vi "Get LabVIEW Install Paths.vi"(8 "Error In":errorcluster) -> (0 "Error Out":errorcluster, 2 "LV Directories":path[](array[path]), 3 "LV Version":string[](array[string]))   [LabVIEW 2014, in "LMH-Toolbox.lvlib"]
doc: "This VI returns the absolute path for each <LabVIEW> directory on the system. \n\nFor example:\nC:\\Program Files (x86)\\National Instruments\\LabVIEW 2011\nC:\\Program Files (x86)\\National Instruments\\LabVIEW 2013"
uses:
  <vilib>/MakerHub/Toolbox/LMH-Toolbox.lvlib
  <vilib>/registry/registry.llb/Registry SAM.ctl
  <vilib>/registry/registry.llb/Read Registry Value Simple STR.vi
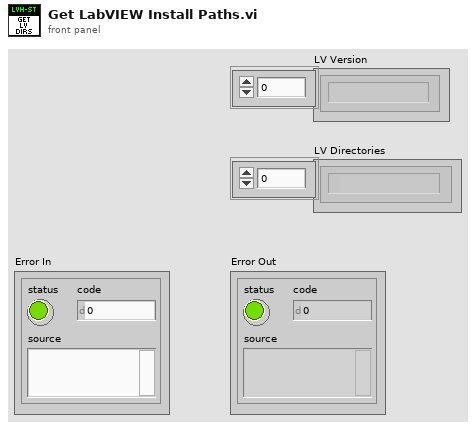
[diagram p1: front panel]
types:
  T1 = typedef "Registry SAM.ctl" = enum32{"KEY_QUERY_VALUE", "KEY_SET_VALUE", "KEY_CREATE_SUB_KEY", "KEY_ENUMERATE_SUB_KEYS", "KEY_NOTIFY", "KEY_CREATE_LINK", "KEY_READ", "KEY_WRITE", "KEY_ALL_ACCESS", "KEY_READ | KEY_WRITE"}
  T2 = typedef "Registry refnum.ctl" = refnum<k1>
  T3 = cluster{"numSubKeys":i32, "maxSubKeyLen":i32, "maxSubKeyClassLen":i32}
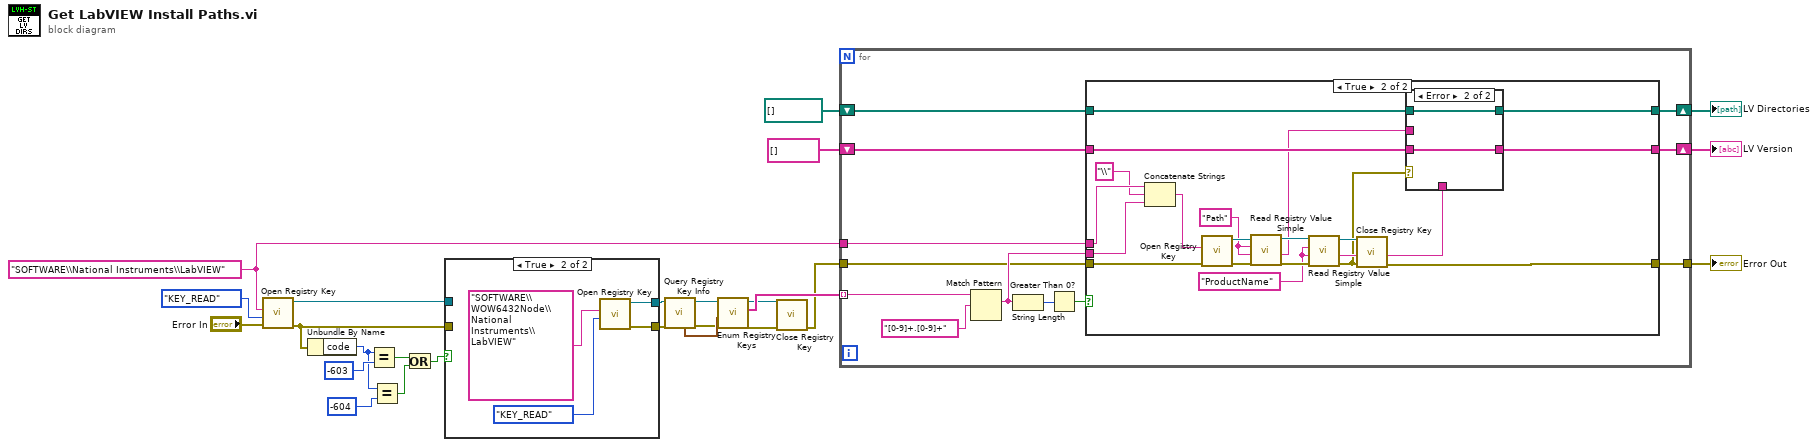
[diagram p0: block diagram]
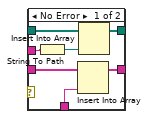
[diagram p4: hidden frame]
diagram:
  w19 = "SOFTWARE\\National Instruments\\LabVIEW" ("subkey")
  n1 = call <vilib>:"Open Registry Key.vi"("error in (no error)"="Error In", "security access mask (KEY_READ | KEY_WRITE)"=Registry_SAM."KEY_READ", "subkey"=w19) -> ("error out"=w10:errorcluster, "refnum out"=w8:T2)  [unwired: 7 in]
  n2 = Unbundle By Name(w10) -> ("code"=w3:i32)
  n3 = Equal?(x=w3, y=-603) -> (x = y?=w5:bool)
  n4 = Equal?(x=w3, y=-604) -> (x = y?=w2:bool)
  n5 = Or(x=w5, y=w2) -> (x .or. y?=w6:bool)
  n6 = case shown="True" w6 {
    tunnel: w10 -> [w26 _]
    tunnel: [w27 w30] -> w9
    tunnel: w8 -> [w27 _]
    tunnel: [w26 w29] -> w7
    frame False {
      # "Found x32 Entry"
    }
    frame True {
      n7 = call <vilib>:"Open Registry Key.vi"("security access mask (KEY_READ | KEY_WRITE)"=Registry_SAM."KEY_READ", "subkey"="SOFTWARE\\WOW6432Node\\National Instruments\\LabVIEW") -> ("error out"=w29:errorcluster, "refnum out"=w30:T2)  [unwired: 8 in]
    }
  }
  n8 = call <vilib>:"Query Registry Key Info.vi"("error in (no error)"=w7, "refnum"=w9) -> ("error out"=w23:errorcluster, "refnum out"=w25:T2, "subkey info"=w24:T3)  [unwired: 5 in, 2 out]
  n9 = call <vilib>:"Enum Registry Keys.vi"("error in (no error)"=w23, "subkey info"=w24, "refnum"=w25) -> ("error out"=w20:errorcluster, "subkeys"=w22:string[], "refnum out"=w21:T2)  [unwired: 6 in]
  n10 = call <vilib>:"Close Registry Key.vi"("error in (no error)"=w20, "refnum"=w21) -> ("error out"=w18:errorcluster)  [unwired: 5 in]
  n11 = for {
    tunnel: w22 -> [w43] mode=indexing
    tunnel: w19 -> [w39]
    shift-right: [w34] -> w14
    shift-left: string[] [] -> [w35]
    shift-right: [w32] -> w12
    shift-left: path[] [] -> [w33]
    tunnel: w18 -> [w37]
    tunnel: [w36] -> w16
    n12 = Match Pattern(string=w43, regular expression="[0-9]+.[0-9]+") -> (match substring=w38:string)  [unwired: 1 in, 3 out]
    n13 = String Length(string=w38) -> (length=w41:i32)
    n14 = Greater Than 0?(x=w41) -> (x > 0?=w40:bool)
    n15 = case shown="True" w40 {
      tunnel: w39 -> [_ w66]
      tunnel: w38 -> [_ w62]
      tunnel: w37 -> [w46 w64]
      tunnel: [w46 w58] -> w36
      tunnel: w35 -> [w44 w53]
      tunnel: [w44 w51] -> w34
      tunnel: w33 -> [w45 w50]
      tunnel: [w45 w49] -> w32
      frame False {
      }
      frame True {
        w54 = "ProductName" ("value")
        w59 = "Path" ("value")
        n16 = Concatenate Strings(w66, "\\" ("string"), w62) -> (w65:string)
        n17 = call <vilib>:"Open Registry Key.vi"("error in (no error)"=w64, "subkey"=w65) -> ("error out"=w60:errorcluster, "refnum out"=w61:T2)  [unwired: 8 in]
        n18 = call-poly <vilib>:"Read Registry Value Simple.vi"("error in (no error)"=w60, "default data"=w59, "value"=w59, "refnum"=w61) -> ("error out"=w57:errorcluster, "String/Binary data"=w48:string, "refnum out"=w56:T2)  [unwired: 2 in, 1 out]
        n19 = call-poly <vilib>:"Read Registry Value Simple.vi"("error in (no error)"=w57, "default data"=w54, "value"=w54, "refnum"=w56) -> ("error out"=w47:errorcluster, "String/Binary data"=w52:string, "refnum out"=w55:T2)  [unwired: 2 in, 1 out]
        n20 = call <vilib>:"Close Registry Key.vi"("error in (no error)"=w47, "refnum"=w55) -> ("error out"=w58:errorcluster)  [unwired: 5 in]
        n21 = case shown="Error" w47 {
          tunnel: w53 -> [w73 w74]
          tunnel: w52 -> [w72 _]
          tunnel: [w71 w74] -> w51
          tunnel: w50 -> [w70 w75]
          tunnel: [w69 w75] -> w49
          tunnel: w48 -> [w68 _]
          frame No Error {
            n22 = String To Path(string=w68) -> (path=w67:path)
            n23 = Insert Into Array(array=w73, new element=w72) -> (w71:string[])  [unwired: 1 in]
            n24 = Insert Into Array(array=w70, new element=w67) -> (w69:path[])  [unwired: 1 in]
          }
          frame Error {
          }
        }
      }
    }
  }
  "Error Out" <- w16
  "LV Version" <- w14
  "LV Directories" <- w12
